vi "FTW-SQLite-ExecuteScript.vi"(0 "SQLite Connection":refnum<data-value>, 5 "SQL Script":string, 11 "error in":errorcluster) -> (4 "SQLite Connection out":refnum<data-value>, 6 "SQL Debug String":string, 15 "error out":errorcluster)   [LabVIEW 2014]
uses:
  core/FTW-SQLite-Core-Structure.ctl
  time/FTW-Time-Uptime.vi
  lib/FTW-LibraryFilepath.vi
  error/FTW-ERR-ThrowGenericError.vi
  error/FTW-ERR-ThrowError.vi
  error/FTW-ERR-CallChain.vi
  string/FTW-STR-ReplaceWhitespace.vi
panel:
  # "Inputs"
  # "Outputs"
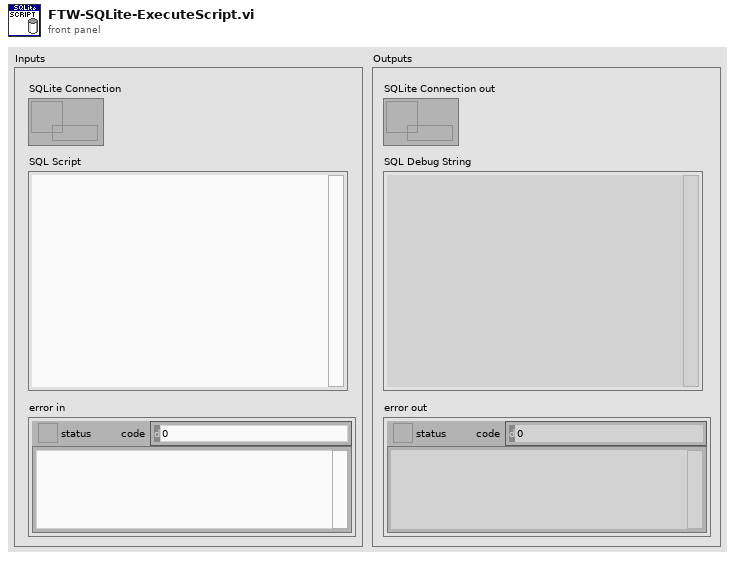
[diagram p1: front panel]
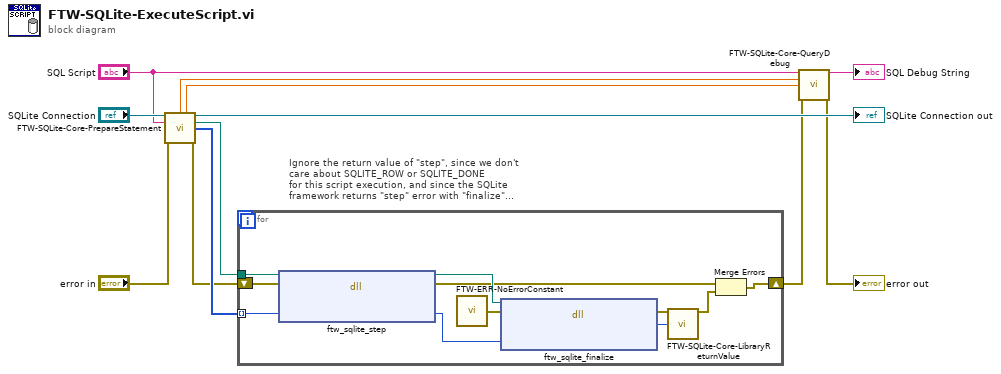
[diagram p0: block diagram]
diagram:
  n1 = call "FTW-SQLite-Core-PrepareStatement.vi"("SQLite Connection"="SQLite Connection", "SQL Statement"="SQL Script", "error in"="error in") -> ("Begin Timestamp"=w2:dbl, "Compile Time"=w1:dbl, "SQLite Connection out"=→"SQLite Connection out":refnum<data-value>, "SQLite Library Filepath"=w9:path, "Prepared Statements"=w10:i64[], "error out"=w8:errorcluster)  [unwired: 7 in]
  n2 = for "Ignore the return value of \"step\", since we don't care about SQLITE_ROW or SQLITE_DONE\nfor this script execution, and since the SQLite framework returns \"step\" error with \"finalize\"\nanyway. Also, we \"finalize\" every prepared statement unconditionally of upstream errors,\nbut only execute \"step\" if no upstream errors." {
    tunnel: w10 -> [w21] mode=indexing
    shift-right: [w15] -> w6
    shift-left: w8 -> [w23]
    tunnel: w9 -> [w22]
    n3 = dll-call lib="?" fn="ftw_sqlite_step"(path in=w22, error in=w23, "Prepared Statement Pointer"=w21) -> (path out=w17:path, error out=w16:errorcluster, "Prepared Statement Pointer"=w20:i64)  [unwired: 2 in]
    n4 = call "FTW-ERR-NoErrorConstant.vi"() -> ("no error"=w13:errorcluster)
    n5 = dll-call lib="?" fn="ftw_sqlite_finalize"(path in=w17, error in=w13, "Prepared Statement Pointer"=w20) -> (error out=w19:errorcluster, "Return Value"=w18:i32)  [unwired: 2 in, 1 out]
    n6 = call "FTW-SQLite-Core-LibraryReturnValue.vi"("error in"=w19, "Return Value"=w18) -> ("error out"=w14:errorcluster)  [unwired: 13 in]
    n7 = Merge Errors(w16, w14) -> (w15:errorcluster)
  }
  n8 = call "FTW-SQLite-Core-QueryDebug.vi"("SQL Script"="SQL Script", "Begin Timestamp"=w2, "Compile Time"=w1, "error in"=w6) -> ("SQL Debug String"=→"SQL Debug String":string, "error out"=→"error out":errorcluster)  [unwired: 10 in]
